vi "ETH12_E3L_waveform.vi"(7 "Waveform":waveform(dbl), 11 "Array in":dbl[](array[numeric])) -> (3 "Array out":waveform(dbl)[](array[waveform]))   [LabVIEW 2022 SP3]
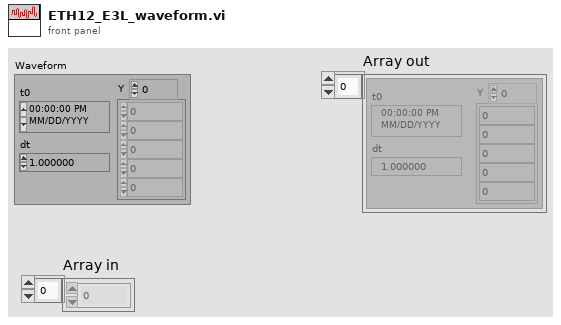
[diagram p1: front panel]
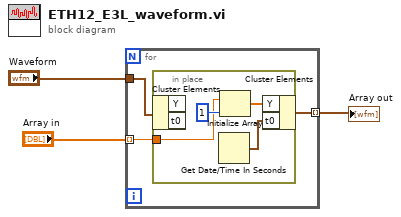
[diagram p0: block diagram]
diagram:
  n1 = for {
    tunnel: [w6] -> w3 mode=indexing
    tunnel: "Waveform" -> [w5]
    tunnel: "Array in" -> [w4] mode=indexing
    n2 = in-place {
      in-place-border: w4 -> [w7]
      n3 = in-place-cluster #1(w5) -> ()  [unwired: 2 out]
      n4 = Get Date/Time In Seconds() -> (seconds since 1Jan1904=w10:timestamp)
      n5 = Initialize Array(w7, 1 ("dimension size")) -> (w9:dbl[])
      n6 = in-place-cluster #1("Y"=w9, "t0"=w10) -> (w6:waveform(dbl))
    }
  }
  "Array out" <- w3
